vi "LedClose (SubVI).vi"(8 "error in (no error)":errorcluster, 11 "LedRef":refnum<class "Digital Output.lvclass">[](array[class])) -> (0 "error out":errorcluster)   [LabVIEW 2020]
uses:
  <vilib>/CISH Robotics/L4VMX VMXpi/Digital Output/Digital Output.lvclass
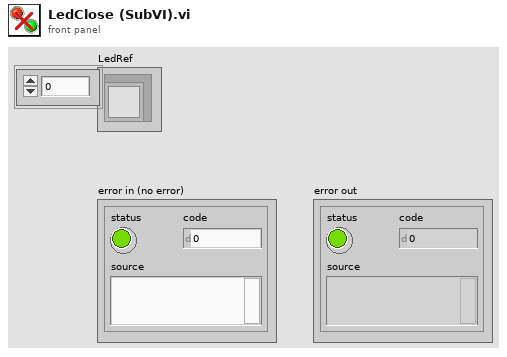
[diagram p1: front panel]
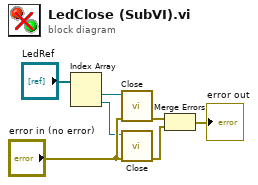
[diagram p0: block diagram]
diagram:
  n1 = Index Array(array="LedRef") -> (element #1=w2:refnum<class "Digital Output.lvclass">, element #2=w3:refnum<class "Digital Output.lvclass">)  [unwired: 2 in]
  n2 = call <vilib>:"Close.vi"("Error In"="error in (no error)", "Digital Output Object"=w2) -> ("Error Out"=w4:errorcluster)  [unwired: 9 in]
  n3 = call <vilib>:"Close.vi"("Error In"="error in (no error)", "Digital Output Object"=w3) -> ("Error Out"=w5:errorcluster)  [unwired: 9 in]
  n4 = Merge Errors(w4, w5) -> (→"error out":errorcluster)
